vi "Configure Measurement (Spectrum Emissions Mask).vi"(0 "VISA resource name":refnum<visa-resource-name>, 1 "Channel Integration Bandwidth (2E+6 Hz)":dbl=2000000.0 format="%#.6g", 2 "Channel Span (5E+6 Hz)":dbl=5000000.0 format="%#.6g", 5 "Measurement Type (0: Total Power Reference)":u16(ring) items=["Total Power Reference", "Power Spectral Density"], 7 "Enable Auto Reference (T: Enable)":bool=TRUE, 9 "Manual Reference (0 dBm)":dbl format="%#.6g", 11 "error in (no error)":errorcluster, 12 "Sweep Time":T2={"Enable Auto Sweep Time (T: Enable)"=TRUE, "Manual Sweep Time (10 ms)"=0.01} {"Manual Sweep Time (10 ms)" format="%#.6g"}, 13 "Resolution Bandwidth":T1={"Enable Auto Resolution Bandwidth (T: Enable)"=TRUE, "Manual Resolution Bandwidth (100000 Hz)"=100000.0} {"Manual Resolution Bandwidth (100000 Hz)" format="%#.6g"}) -> (4 "VISA resource name out":refnum<visa-resource-name>, 15 "error out":errorcluster)   [LabVIEW 2014, in "Agilent ESA PSA Series.lvlib"]
doc: "Sets up the spectrum emissions measurement."
uses:
  Agilent ESA PSA Series.lvlib
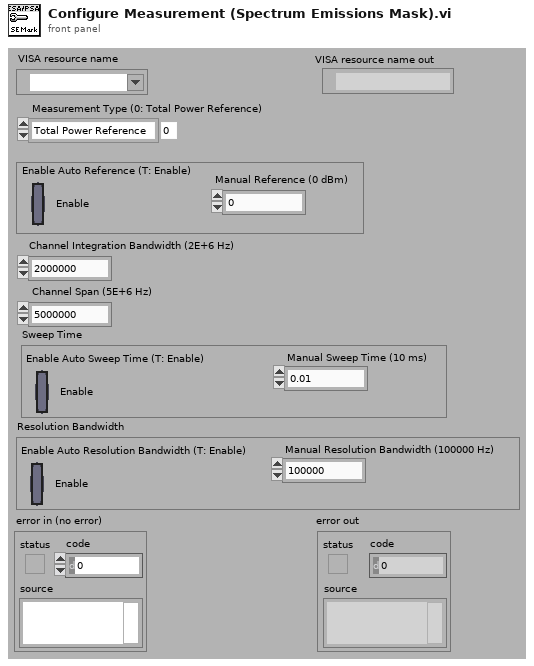
[diagram p1: front panel]
types:
  T1 = cluster{"Enable Auto Resolution Bandwidth (T: Enable)":bool, "Manual Resolution Bandwidth (100000 Hz)":dbl}
  T2 = cluster{"Enable Auto Sweep Time (T: Enable)":bool, "Manual Sweep Time (10 ms)":dbl}
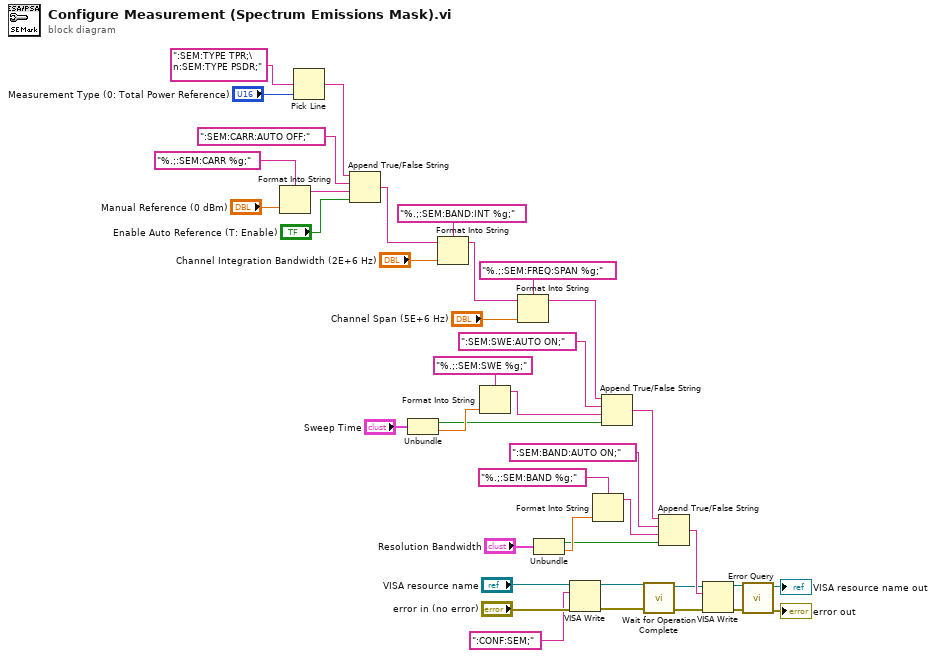
[diagram p0: block diagram]
diagram:
  n1 = Format Into String(format string="%.;:SEM:CARR %g;", "Manual Reference (0 dBm)") -> (resulting string=w34:string)  [unwired: 2 in, 1 out]
  n2 = Pick Line(multi-line string=":SEM:TYPE TPR;\n:SEM:TYPE PSDR;" ("format string"), line index="Measurement Type (0: Total Power Reference)") -> (output string=w10:string)  [unwired: 1 in]
  n3 = Append True/False String(1:"Enable Auto Reference (T: Enable)", 2:w34, 3:":SEM:CARR:AUTO OFF;" ("true string"), 4:w10) -> (0:w11:string)
  n4 = Unbundle("Sweep Time") -> ("Enable Auto Sweep Time (T: Enable)"=w26:bool, "Manual Sweep Time (10 ms)"=w28:dbl)
  n5 = Format Into String(format string="%.;:SEM:BAND:INT %g;", initial string=w11, "Channel Integration Bandwidth (2E+6 Hz)") -> (resulting string=w12:string)  [unwired: 1 in, 1 out]
  n6 = Format Into String(format string="%.;:SEM:SWE %g;", w28) -> (resulting string=w25:string)  [unwired: 2 in, 1 out]
  n7 = Format Into String(format string="%.;:SEM:FREQ:SPAN %g;", initial string=w12, "Channel Span (5E+6 Hz)") -> (resulting string=w13:string)  [unwired: 1 in, 1 out]
  n8 = Unbundle("Resolution Bandwidth") -> ("Enable Auto Resolution Bandwidth (T: Enable)"=w20:bool, "Manual Resolution Bandwidth (100000 Hz)"=w22:dbl)
  n9 = VISA Write(VISA resource name="VISA resource name", write buffer=":CONF:SEM;" ("string (\"\")"), error in (no error)="error in (no error)") -> (VISA resource name out=w6:refnum<visa-resource-name>, error out=w7:errorcluster)  [unwired: 1 out]
  n10 = Format Into String(format string="%.;:SEM:BAND %g;", w22) -> (resulting string=w18:string)  [unwired: 2 in, 1 out]
  n11 = Append True/False String(1:w26, 2:w25, 3:":SEM:SWE:AUTO ON;" ("initial string"), 4:w13) -> (0:w14:string)
  n12 = call "Wait for Operation Complete.vi"("error in (no error)"=w7, "VISA resource name"=w6) -> ("error out"=w4:errorcluster, "VISA resource name out"=w5:refnum<visa-resource-name>)  [unwired: 8 in]
  n13 = Append True/False String(1:w20, 2:w18, 3:":SEM:BAND:AUTO ON;" ("initial string"), 4:w14) -> (0:w15:string)
  n14 = VISA Write(VISA resource name=w5, write buffer=w15, error in (no error)=w4) -> (VISA resource name out=w9:refnum<visa-resource-name>, error out=w8:errorcluster)  [unwired: 1 out]
  n15 = call "Error Query.vi"("error in (no error)"=w8, "VISA resource name"=w9) -> ("error out"=→"error out":errorcluster, "VISA resource name out"=→"VISA resource name out":refnum<visa-resource-name>)  [unwired: 6 in, 2 out]
